vi "Unmarshal.vi"(8 "error in (no error)":errorcluster, 10 "Buffer":u8[](array[numeric]), 11 "int32 in":refnum<class "bytes.lvclass">) -> (0 "error out":errorcluster, 2 "Buffer Count":i32=8, 3 "int32 out":refnum<class "bytes.lvclass">)   [LabVIEW 2020, in "Protobuf RAW.lvlib" / "bytes.lvclass"]
uses:
  bytes.lvclass
  bytes.lvclass/bytes.ctl
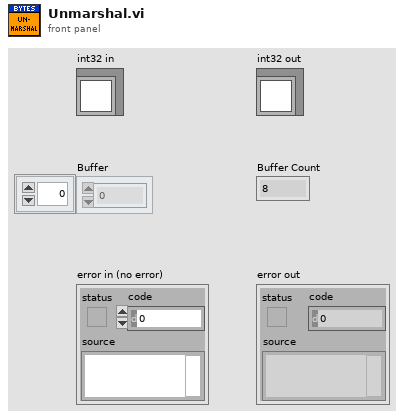
[diagram p1: front panel]
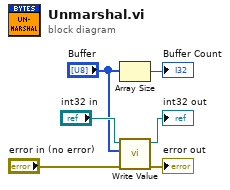
[diagram p0: block diagram]
diagram:
  n1 = Array Size(array="Buffer") -> (size(s)=→"Buffer Count":i32)
  n2 = call "Write Value.vi"("error in (no error)"="error in (no error)", "Value"="Buffer", "fixed32 in"="int32 in") -> ("error out"=→"error out":errorcluster, "fixed32 out"=→"int32 out":refnum<class "bytes.lvclass">)  [unwired: 7 in]
